vi "Global.vi"() -> ()   [LabVIEW 2011]
panel:
  out "Encoder BL":string
  out "Encoder FL":string
  out "Encoder BR":string
  out "Encoder FR":string
  out "DriveMotors":string
  out "PivotMotors":string
  out "Joystick 2":string
  out "Joystick 1":string
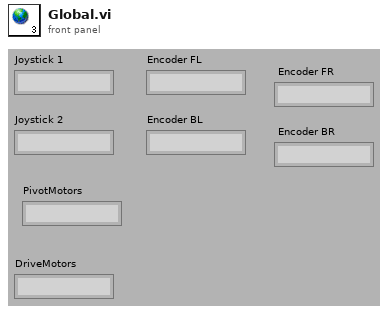
[diagram p1: front panel]
diagram:
